vi "OAuth2 Error Message.vi"(5 "Redirect URI":refnum<class "URI.lvclass">, 7 "Requested Scopes":string[](array[string]), 10 "OAuth2 Error":T1) -> (2 "Error Message":string)   [LabVIEW 2020, in "OAuth2.lvlib"]
uses:
  OAuth2.lvlib
  OAuth2 Error.ctl
  <vilib>/IlluminatedG/lv-stream/URI/URI.lvclass
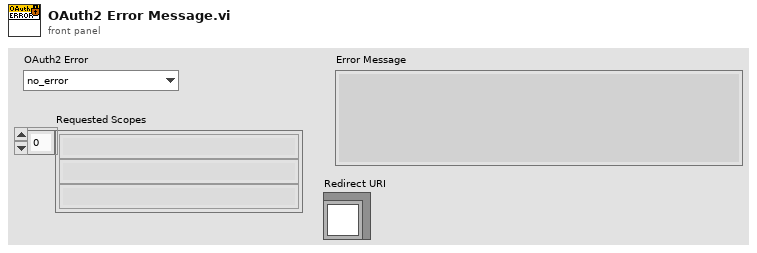
[diagram p1: front panel]
types:
  T1 = typedef "OAuth2.lvlib/OAuth2 Error.ctl" = enum16{"no_error", "admin_policy_enforced", "disallowed_useragent", "org_internal", "invalid_grant", "redirect_uri_mismatch"}
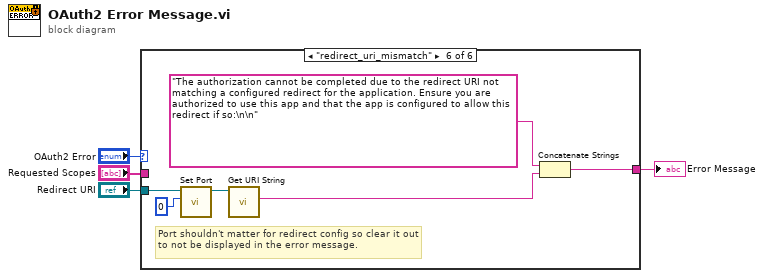
[diagram p0: block diagram]
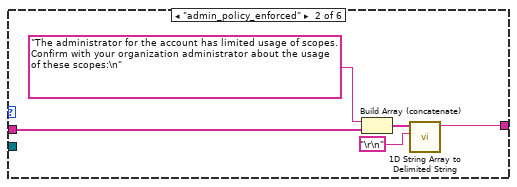
[diagram p3: hidden frame]
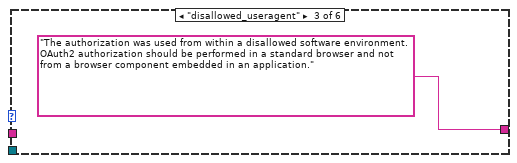
[diagram p4: hidden frame]
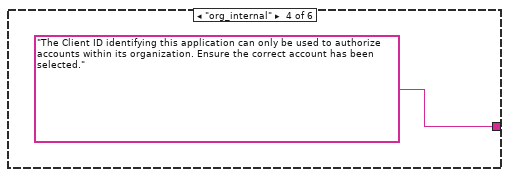
[diagram p5: hidden frame]
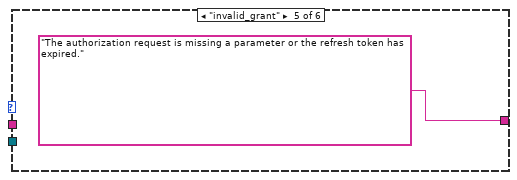
[diagram p6: hidden frame]
diagram:
  n1 = case shown="\"redirect_uri_mismatch\"" "OAuth2 Error" {
    tunnel: "Requested Scopes" -> [_ w9 _ _ _ _]
    tunnel: [_ w5 "The authorization was used from within a disallowed software environment. OAuth2 authorization should be performed in a standard browser and not from a browser component embedded in an application." "The Client ID identifying this application can only be used to authorize accounts within its organization. Ensure the correct account has been selected." "The authorization request is missing a parameter or the refresh token has expired." w13] -> w2
    tunnel: "Redirect URI" -> [_ _ _ _ _ w18]
    frame "no_error" {
    }
    frame "admin_policy_enforced" {
      n2 = Build Array (concatenate)("The administrator for the account has limited usage of scopes. Confirm with your organization administrator about the usage of these scopes:\n", w9) -> (w7:string[])
      n3 = call <vilib>:"1D String Array to Delimited String.vi"("delimiter"="\r\n", "string array"=w7) -> ("delimited string"=w5:string)  [unwired: 9 in]
    }
    frame "disallowed_useragent" {
    }
    frame "org_internal" {
    }
    frame "invalid_grant" {
    }
    frame "redirect_uri_mismatch" {
      # "Port shouldn't matter for redirect config so clear it out to not be displayed in the error message."
      n4 = call <vilib>:"Set Port.vi"("Port"=u16 0, "URI in"=w18) -> ("URI out"=w16:refnum<class "URI.lvclass">)  [unwired: 8 in, 1 out]
      n5 = call <vilib>:"Get URI String.vi"("URI in"=w16) -> ("URI String"=w14:string)  [unwired: 8 in, 2 out]
      n6 = Concatenate Strings("The authorization cannot be completed due to the redirect URI not matching a configured redirect for the application. Ensure you are authorized to use this app and that the app is configured to allow this redirect if so:\n\n", w14) -> (w13:string)
    }
  }
  "Error Message" <- w2
